vi "Update Card.vi"(8 "error in (no error)":errorcluster, 11 "BME_DG_G05_Chnl in":refnum<class "BME_DG_G05_Chnl.lvclass">) -> (0 "error out":errorcluster, 3 "BME_DG_G05_Chnl out":refnum<class "BME_DG_G05_Chnl.lvclass">)   [LabVIEW 2009, in "BME_DG_G05_Chnl.lvclass"]
uses:
  BME_DG_G05_Chnl.lvclass
  LV-BME Interface/ChnlWithModulo.ctl
  BME_DG_G05_Chnl.lvclass/BME_DG_G05_Chnl.ctl
panel:
  in  "ChnParameter":T1={" Delay (µs)"=0.0, "TriggerModulo"=1, "On? (false)"=FALSE, "PositiveVoltage?(true)"=FALSE, "50OhmTerminated? "=FALSE, "25OhmOutput?"=FALSE} {"TriggerModulo" min=1 max=1000000; "Delay (µs)" min=0.0 max=100000000.0 format="%.5f"}
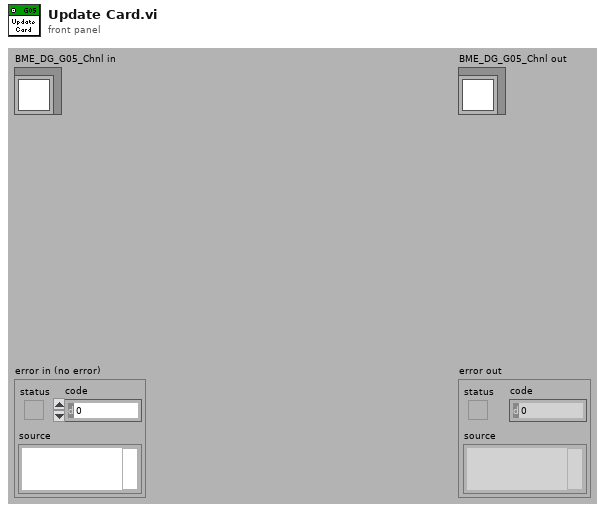
[diagram p1: front panel]
types:
  T1 = typedef "ChnlWithModulo.ctl" = cluster{" Delay (µs)":dbl, "TriggerModulo":u32, "On? (false)":bool, "PositiveVoltage?(true)":bool, "50OhmTerminated? ":bool, "25OhmOutput?":bool}
  T2 = typedef "ChnlSettings.ctl" = cluster{" Delay (µs)":dbl, "On? (false)":bool, "PositiveVoltage?(true)":bool, "50OhmTerminated? ":bool, "25OhmOutput?":bool}
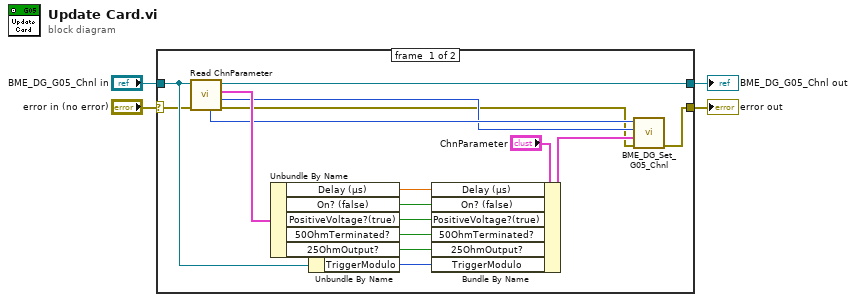
[diagram p0: block diagram]
diagram:
  n1 = case shown="No Error" "error in (no error)" {
    selector: "error in (no error)" -> [w7 w22]
    tunnel: [w5 w22] -> w1
    tunnel: [w20 w21] -> w3
    tunnel: "BME_DG_G05_Chnl in" -> [w11 w21]
    frame #0 {
      n2 = call-dynamic "Read ChnParameter.vi"("error in (no error)"=w7, "BME_DG_Chnl in"=w11) -> ("error out"=w6:errorcluster, "Nr"=w8:i32, "ChnParemater"=w17:T2, "BME_DG_Chnl out"=w20:refnum<class "BME_DG_G05_Chnl.lvclass">, "DG Nr"=w9:i32)  [unwired: 4 in, 1 out]
      n3 = Unbundle By Name(w17) -> ("Delay (µs)"=w16:dbl, "On? (false)"=w15:bool, "PositiveVoltage?(true)"=w14:bool, "50OhmTerminated?"=w13:bool, "25OhmOutput?"=w12:bool)
      n4 = Unbundle By Name(w11) -> ("TriggerModulo"=w10:i32)
      n5 = Bundle By Name(cluster="ChnParameter", "Delay (µs)"=w16, "On? (false)"=w15, "PositiveVoltage?(true)"=w14, "50OhmTerminated?"=w13, "25OhmOutput?"=w12, "TriggerModulo"=w10) -> (w18:T1)
      n6 = call "BME_DG_Set_G05_Chnl.vi"("error in (no error)"=w6, "ChnParemater"=w18, "Channel"=w8, "DG_Number"=w9) -> ("error out"=w5:errorcluster)  [unwired: 6 in, 1 out]
    }
    frame #1 {
    }
  }
  "error out" <- w1
  "BME_DG_G05_Chnl out" <- w3
